vi "Get Config Log.vi"(8 "error in (no error)":errorcluster, 10 "Parse All":bool, 11 "Plugin Manager in":refnum<class "CIFPluginManager.lvclass">) -> (0 "error out":errorcluster, 2 "Filtered Config Entries":string, 3 "Plugin Manager out":refnum<class "CIFPluginManager.lvclass">)   [LabVIEW 2021, in "CIFPluginManager.lvclass"]
uses:
  CIFPluginManager.lvclass
  CIFPluginManager.lvclass/CIFPluginManager.ctl
  CIFUtilities/CIFLogs/CIFLogs.lvlib
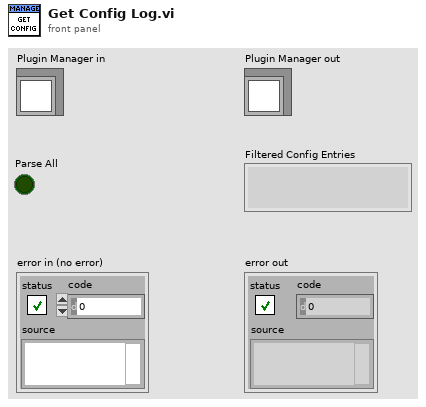
[diagram p1: front panel]
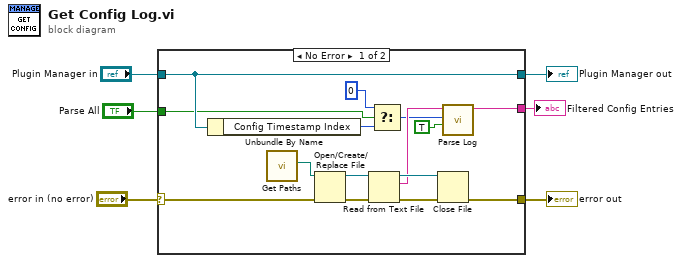
[diagram p0: block diagram]
diagram:
  n1 = case shown="No Error" "error in (no error)" {
    selector: "error in (no error)" -> [w19 w23]
    tunnel: [w16 w23] -> w5
    tunnel: [w15 w22] -> w3
    tunnel: "Plugin Manager in" -> [w15 w22]
    tunnel: [w8 _] -> w1
    tunnel: "Parse All" -> [w12 _]
    frame No Error {
      n2 = Unbundle By Name(w15) -> ("Config Timestamp Index"=w14:u64)
      n3 = call "Get Paths.vi"() -> ("Config Log"=w10:path)  [unwired: 9 in, 2 out]
      n4 = Open/Create/Replace File(file path (use dialog)=w10, error in=w19) -> (refnum out=w20:refnum<file>, error out=w18:errorcluster)  [unwired: 4 in, 1 out]
      n5 = Read from Text File(file (use dialog)=w20, error in=w18) -> (refnum out=w21:refnum<file>, text=w11:string, error out=w17:errorcluster)  [unwired: 2 in, 1 out]
      n6 = Select(t=u64 0, s=w12, f=w14) -> (s? t:f=w9:u64)
      n7 = Close File(refnum=w21, error in=w17) -> (error out=w16:errorcluster)  [unwired: 1 out]
      n8 = call "Parse Log.vi"("Strip Timestamp"=TRUE, "Index Timestamp"=w9, "Log"=w11) -> ("Filtered Config Entries"=w8:string)  [unwired: 8 in]
    }
    frame Error {
    }
  }
  "error out" <- w5
  "Plugin Manager out" <- w3
  "Filtered Config Entries" <- w1
